vi "Commascript advanced.vi"() -> ()   [LabVIEW 2017]
panel:
  out "Height":u32
  out "Width":u32
  out "Scaling Factor":dbl=1.07143 format="%#_13g"
  out "concatenated string":string
  out "stripped path":path
  out "appended path":path
  out "stripped path 2":path
  in  "Starting Pos":i16(slide)=128 scale=340.0..50.0
  in  "string":string
  out "new picture":picture
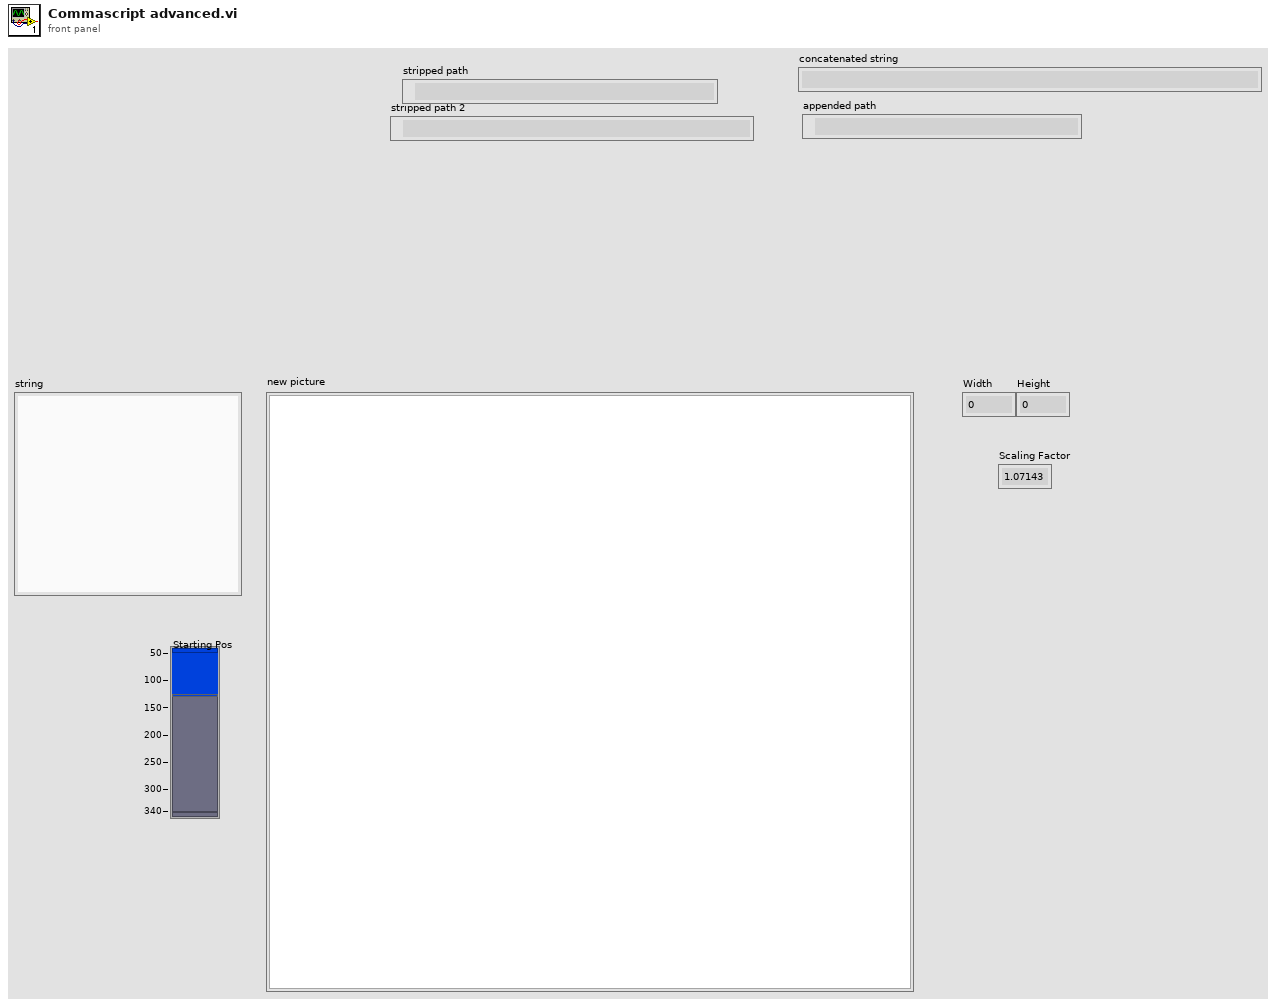
[diagram p1: front panel]
types:
  T1 = enum32{"invalid app kind", "Development System", "Run Time System", "Student Edition", "Embedded LabVIEW", "Evaluation", "Custom"}
  T2 = typedef "imagedata.ctl" = cluster{"image type":i32, "image depth":i32, "image":u8[], "mask":u8[], "colors":u32[], "Rectangle":cluster{"left":i16, "top":i16, "right":i16, "bottom":i16}}
  T3 = typedef "LVBoundsTypeDef.ctl" = cluster{"Width":u32, "Height":u32}
  T4 = cluster{"Width":u16, "Style":enum32{"Solid", "Dash", "Dot", "DashDot", "DashDotDot"}}
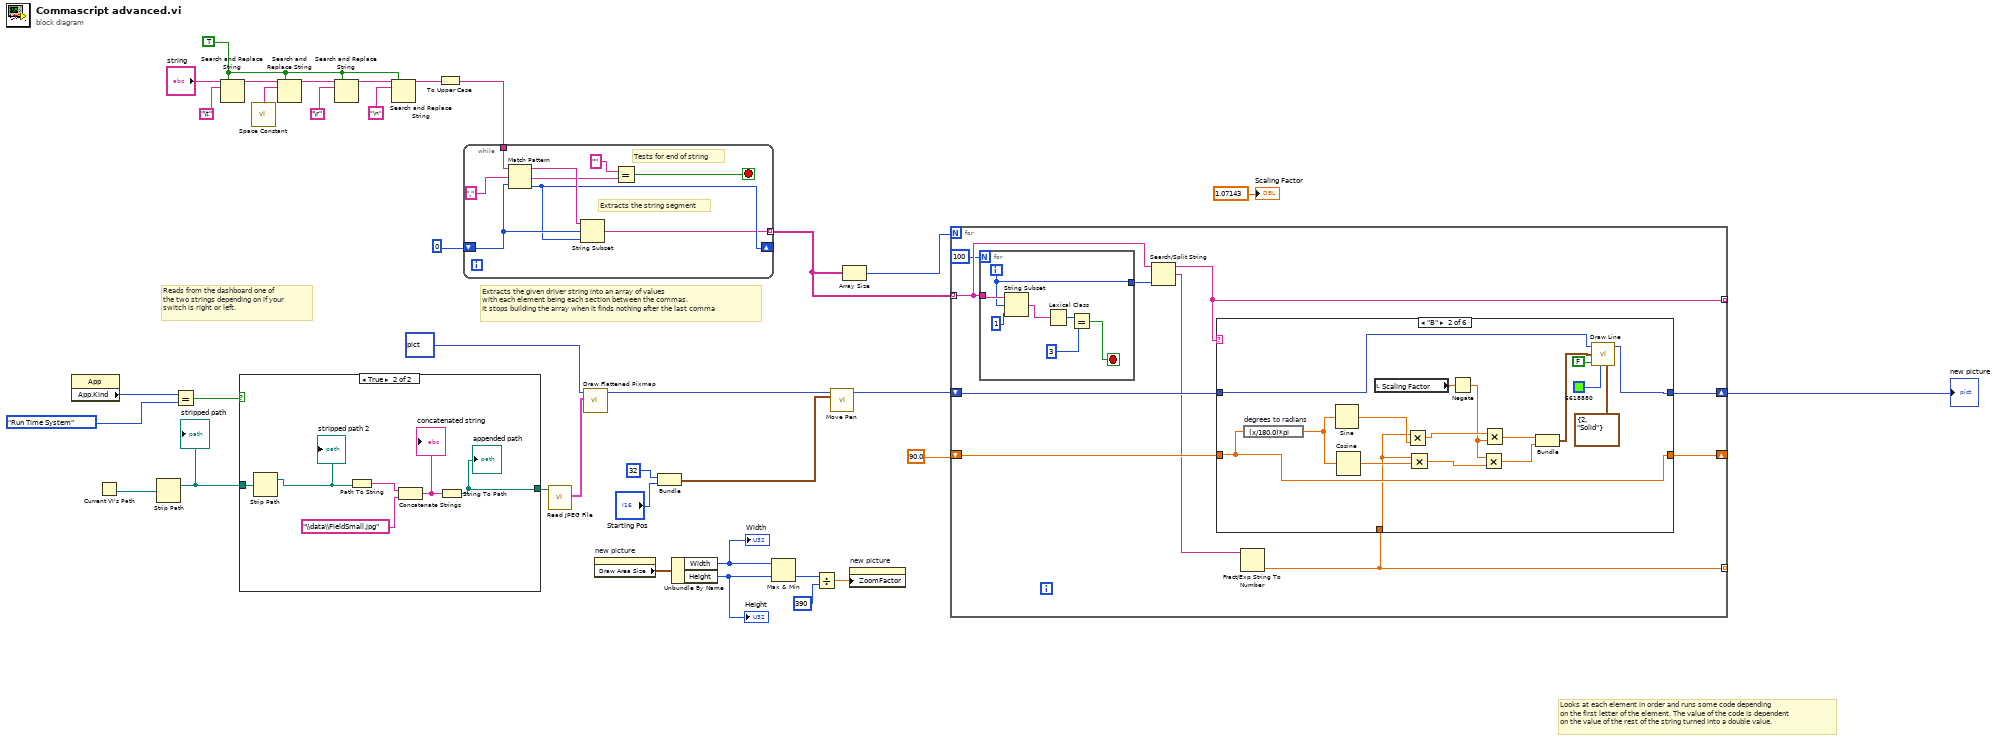
[diagram p0: block diagram]
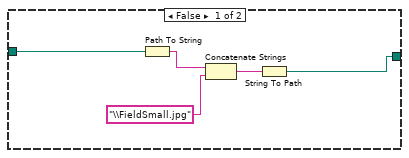
[diagram p2: hidden frame]
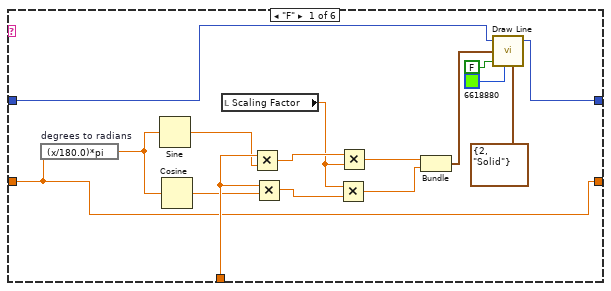
[diagram p3: hidden frame]
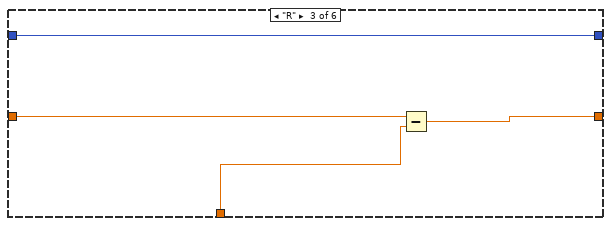
[diagram p4: hidden frame]
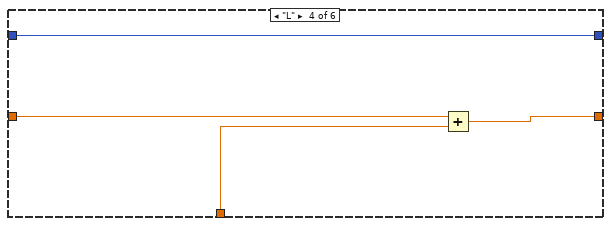
[diagram p5: hidden frame]
diagram:
  w18 = TRUE ("replace all? (F)")
  # "Reads from the dashboard one of\nthe two strings depending on if your\nswitch is right or left."
  # "Extracts the given driver string into an array of values \nwith each element being each section between the commas.\nIt stops building the array when it finds nothing after the last comma"
  # "Looks at each element in order and runs some code depending\non the first letter of the element. The value of the code is dependent\non the value of the rest of the string turned into a double value."
  n1 = property class="App"() -> ("App.Kind"=w12:T1)  [unwired: 2 in, 2 out]
  n2 = Current VI's Path() -> (path=w15:path)
  n3 = Strip Path(path=w15) -> (stripped path=w14:path)  [unwired: 1 out]
  "stripped path" <- w14
  n4 = Equal?(x=w12, y=T1."Run Time System") -> (x = y?=w10:bool)
  n5 = Search and Replace String(replace all?=w18, input string="string", search string="\t") -> (result string=w23:string)  [unwired: 5 in, 3 out]
  n6 = case shown="True" w10 {
    tunnel: w14 -> [w39 w47]
    tunnel: [w37 w42] -> w9
    frame False {
      n7 = Path To String(path=w39) -> (string=w38:string)
      n8 = Concatenate Strings(w38, "\\FieldSmall.jpg" ("name or relative path")) -> (w41:string)
      n9 = String To Path(string=w41) -> (path=w37:path)
    }
    frame True {
      n10 = Strip Path(path=w47) -> (stripped path=w46:path)  [unwired: 1 out]
      "stripped path 2" <- w46
      n11 = Path To String(path=w46) -> (string=w45:string)
      n12 = Concatenate Strings(w45, "\\data\\FieldSmall.jpg" ("name or relative path")) -> (w43:string)
      "concatenated string" <- w43
      n13 = String To Path(string=w43) -> (path=w42:path)
      "appended path" <- w42
    }
  }
  n14 = call <vilib>:"Space Constant.vi"() -> ("String"=w20:string)
  n15 = Search and Replace String(replace all?=w18, input string=w23, search string=w20) -> (result string=w24:string)  [unwired: 5 in, 3 out]
  n16 = Search and Replace String(replace all?=w18, input string=w24, search string="\r") -> (result string=w25:string)  [unwired: 5 in, 3 out]
  n17 = Search and Replace String(replace all?=w18, input string=w25, search string="\n") -> (result string=w17:string)  [unwired: 5 in, 3 out]
  n18 = To Upper Case(1:w17) -> (0:w16:string)
  n19 = while {
    shift-right: [w53] -> _
    shift-left: 0 ("offset past match") -> [w54]
    tunnel: [w52] -> w26 mode=indexing
    tunnel: w16 -> [w48]
    stop <- w49 stop-if-true
    # "Tests for end of string"
    # "Extracts the string segment"
    n20 = Match Pattern(string=w48, regular expression=",", offset (0)=w54) -> (before substring=w55:string, after substring=w51:string, offset past match=w53:i32)  [unwired: 1 out]
    n21 = String Subset(string=w55, offset (0)=w54, length (rest)=w53) -> (substring=w52:string)
    n22 = Equal?(x="", y=w51) -> (x = y?=w49:bool)
  }
  n23 = call <vilib>:"Read JPEG File.vi"("path to JPEG file"=w9) -> ("image data"=w8:T2)  [unwired: 8 in, 2 out]
  n24 = call <vilib>:"Draw Flattened Pixmap.vi"("image data"=w8, "picture"=picture data[5B]) -> ("new picture"=w31:picture)  [unwired: 7 in]
  n25 = property on="new picture" class="Pict"() -> ("Draw Area Size"=w7:T3)  [unwired: 2 in, 2 out]
  n26 = Bundle("x"=i16 32, "Starting Pos"="Starting Pos") -> (w29:cluster{"x":i16, "Starting Pos":i16})  [unwired: 1 in]
  n27 = Unbundle By Name(w7) -> ("Width"=w5:u32, "Height"=w4:u32)
  "Width" <- w5
  "Height" <- w4
  n28 = Max & Min(x=w5, y=w4) -> (min(x,y)=w3:u32)  [unwired: 1 out]
  n29 = Divide(x=w3, y=u32 390) -> (x/y=w1:dbl)
  n30 = call <vilib>:"Move Pen.vi"("new position"=w29, "picture"=w31) -> ("new picture"=w35:picture)  [unwired: 3 in]
  n31 = Array Size(array=w26) -> (size(s)=w36:i32)
  n32 = property on="new picture" class="Pict"("ZoomFactor"=w1) -> ()  [unwired: 2 in, 2 out]
  n33 = for {
    N: w36 -> [_]
    tunnel: [w66] -> _ mode=indexing
    tunnel: [w59] -> _ mode=indexing
    tunnel: w26 -> [w60] mode=indexing
    shift-right: [w64] -> w33
    shift-left: w35 -> [w65]
    shift-right: [w62] -> _
    shift-left: 90.0 -> [w63]
    n34 = for {
      N: 100 -> [_]
      tunnel: w60 -> [w71]
      tunnel: [w68] -> w61
      i -> [w68]
      stop <- w67 stop-if-true
      n35 = String Subset(string=w71, offset (0)=w68, length (rest)=1 ("length (rest)")) -> (substring=w69:string)
      n36 = Lexical Class(1:w69) -> (0:w73:i16)
      n37 = Equal?(x=w73, y=i16 3) -> (x = y?=w67:bool)
    }
    n38 = Search/Split String(string=w60, offset (0)=w61) -> (substring before match=w59:string, match + rest of string=w58:string)  [unwired: 1 in, 1 out]
    n39 = Fract/Exp String To Number(string=w58) -> (number=w66:dbl)  [unwired: 3 in, 1 out]
    n40 = case shown="\"B\"" w59 {
      tunnel: w66 -> [w86 w98 w107 w111 _ _]
      tunnel: w65 -> [w88 w101 w110 w114 w116 w118]
      tunnel: [w87 w100 w110 w114 w116 w118] -> w64
      tunnel: w63 -> [w82 w99 w108 w112 w115 w117]
      tunnel: [w82 w99 w109 w113 w115 w117] -> w62
      frame "F" {
        n41 = expression code="(x/180.0)*pi" "degrees to radians"(w82) -> (w85:dbl)
        n42 = Sine(x=w85) -> (sin(x)=w83:dbl)
        n43 = Cosine(x=w85) -> (cos(x)=w84:dbl)
        n44 = local read "Scaling Factor"() -> (w74:dbl)
        n45 = Multiply(x=w86, y=w83) -> (x*y=w77:dbl)
        n46 = Multiply(x=w86, y=w84) -> (x*y=w78:dbl)
        n47 = Multiply(x=w74, y=w78) -> (x*y=w75:dbl)
        n48 = Multiply(x=w77, y=w74) -> (x*y=w76:dbl)
        n49 = Bundle(w76, w75) -> (w79:cluster{dbl, dbl})  [unwired: 1 in]
        n50 = call <vilib>:"Draw Line.vi"("picture"=w88, "end point"=w79, "absolute coordinates?(T)"=FALSE, "color(black)"=u32 6618880, "pen"=T4 {"Width"=2, "Style"=enum."Solid"}) -> ("new picture"=w87:picture)  [unwired: 4 in]
      }
      frame "B" {
        n51 = expression code="(x/180.0)*pi" "degrees to radians"(w99) -> (w104:dbl)
        n52 = Sine(x=w104) -> (sin(x)=w102:dbl)
        n53 = Cosine(x=w104) -> (cos(x)=w103:dbl)
        n54 = local read "Scaling Factor"() -> (w91:dbl)
        n55 = Multiply(x=w98, y=w102) -> (x*y=w95:dbl)
        n56 = Multiply(x=w98, y=w103) -> (x*y=w94:dbl)
        n57 = Negate(x=w91) -> (-x=w90:dbl)
        n58 = Multiply(x=w90, y=w94) -> (x*y=w93:dbl)
        n59 = Multiply(x=w95, y=w90) -> (x*y=w92:dbl)
        n60 = Bundle(w92, w93) -> (w105:cluster{dbl, dbl})  [unwired: 1 in]
        n61 = call <vilib>:"Draw Line.vi"("picture"=w101, "end point"=w105, "absolute coordinates?(T)"=FALSE, "color(black)"=u32 6618880, "pen"=T4 {"Width"=2, "Style"=enum."Solid"}) -> ("new picture"=w100:picture)  [unwired: 4 in]
      }
      frame "R" {
        n62 = Subtract(x=w108, y=w107) -> (x-y=w109:dbl)
      }
      frame "L" {
        n63 = Add(x=w112, y=w111) -> (x+y=w113:dbl)
      }
      frame "D", Default {
      }
      frame "IF" {
      }
    }
  }
  "new picture" <- w33
  "Scaling Factor" <- 1.07143 ("Scaling Factor")
